vi "Set Packet Length (bytes).vi"(8 "error in (no error)":errorcluster, 10 "Packet Length ,bytes":i32, 11 "niDTS BT Dut in":refnum<class "niDTS BT Dut.lvclass">) -> (0 "error out":errorcluster, 3 "niDTS BT Dut out":refnum<class "niDTS BT Dut.lvclass">)   [LabVIEW 2015, in "niDTS BT.lvlib" / "niDTS BT Dut.lvclass"]
uses:
  niDTS BT Dut.lvclass
  niDTS BT Dut.lvclass/niDTS BT Dut.ctl
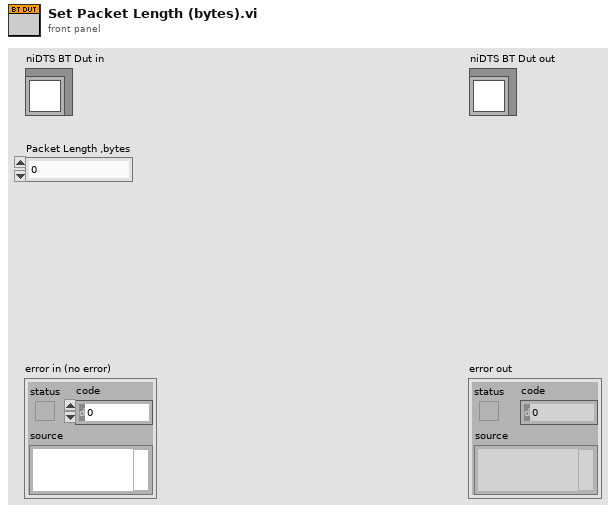
[diagram p1: front panel]
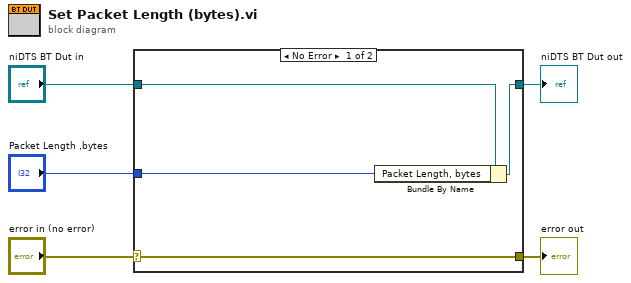
[diagram p0: block diagram]
diagram:
  n1 = case shown="No Error" "error in (no error)" {
    selector: "error in (no error)" -> [w9 w10]
    tunnel: [w9 w10] -> w4
    tunnel: [w7 w11] -> w2
    tunnel: "niDTS BT Dut in" -> [w8 w11]
    tunnel: "Packet Length ,bytes" -> [w6 _]
    frame No Error {
      n2 = Bundle By Name(cluster=w8, "Packet Length, bytes"=w6) -> (w7:refnum<class "niDTS BT Dut.lvclass">)
    }
    frame Error {
    }
  }
  "error out" <- w4
  "niDTS BT Dut out" <- w2
